vi "PH_SHS_Analysis.evt call Set Consider Tilt.vi"(0 "i ref in":refnum<vi>, 1 "Instance":string, 2 "Consider Tilt":bool, 5 "error in (no error)":errorcluster) -> (14 "i ref out":refnum<vi>, 19 "error out":errorcluster)   [LabVIEW 2014, in "PH_SHS_Analysis.lvlib"]
doc: "This VI calls the event case \"ConsiderTilt\" by a simple call."
uses:
  PH_SHS_Analysis.lvlib
  CSCore/CSSystem/CoreLib/CoreLib.short 2 byte array.vi
  CSCore/CSSystem/CoreLib/CoreLib.lvlib
  CSCore/BaseProcess/BaseProcess.lvlib
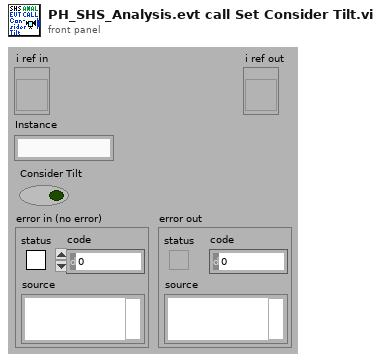
[diagram p1: front panel]
types:
  T1 = typedef "CoreDefs.rawDataType.ctl" = i8[]
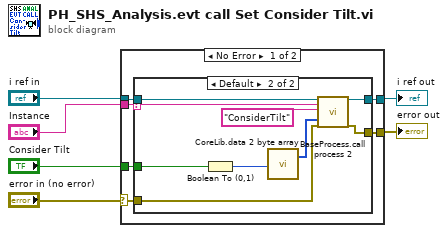
[diagram p0: block diagram]
diagram:
  n1 = case shown="No Error" "error in (no error)" {
    selector: "error in (no error)" -> [w9 w24]
    tunnel: [w12 w25] -> w2
    tunnel: [w11 w24] -> w1
    tunnel: "i ref in" -> [w10 w25]
    tunnel: "Instance" -> [w8 _]
    tunnel: "Consider Tilt" -> [w7 _]
    frame No Error {
      n2 = case shown="Default" w8 {
        selector: w8 -> [_ w17]
        tunnel: [w14 w22] -> w12
        tunnel: [w13 w21] -> w11
        tunnel: w10 -> [w14 w20]
        tunnel: w9 -> [w13 w18]
        tunnel: w7 -> [_ w16]
        frame "N/A" {
        }
        frame Default {
          n3 = Boolean To (0,1)(Boolean=w16) -> (0, 1=w15:i16)
          n4 = call-poly "CoreLib.data 2 byte array.vi"("i16"=w15) -> ("byteArray out"=w19:T1)  [unwired: 18 in]
          n5 = call "BaseProcess.call process 2.vi"("i ref in"=w20, "Object"=w17, "Selector"="ConsiderTilt", "Data"=w19, "error in (no error)"=w18) -> ("i ref out"=w22:refnum<vi>, "error out"=w21:errorcluster)  [unwired: 13 in]
        }
      }
    }
    frame Error {
    }
  }
  "i ref out" <- w2
  "error out" <- w1
